vi "RT_DMARS (SubVI).vi"(5 "y2":dbl[](array[numeric]), 7 "y1":dbl[](array[numeric]), 10 "u8":dbl[](array[numeric]), 11 "u7":dbl[](array[numeric])) -> (3 "DMARS Data":dbl[](array[numeric]))   [LabVIEW 2017]
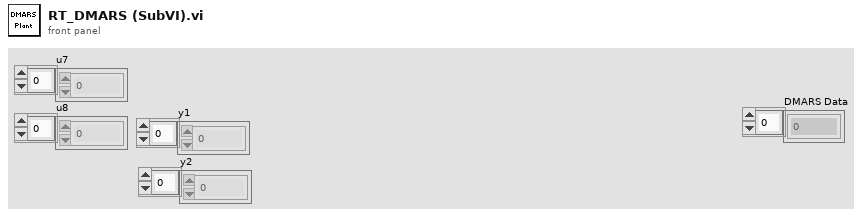
[diagram p1: front panel]
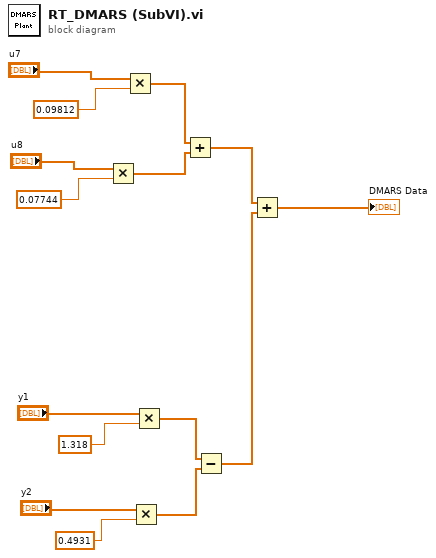
[diagram p0: block diagram]
diagram:
  n1 = Multiply(x="u8", y=0.07744) -> (x*y=w1:dbl[])
  n2 = Multiply(x="u7", y=0.09812) -> (x*y=w7:dbl[])
  n3 = Multiply(x="y2", y=0.4931) -> (x*y=w12:dbl[])
  n4 = Multiply(x="y1", y=1.318) -> (x*y=w13:dbl[])
  n5 = Add(x=w7, y=w1) -> (x+y=w6:dbl[])
  n6 = Subtract(x=w13, y=w12) -> (x-y=w10:dbl[])
  n7 = Add(x=w6, y=w10) -> (x+y=→"DMARS Data":dbl[])
